vi "TCPReadU8.vi"(8 "error in (no error)":errorcluster, 9 "timeout ms (25000)":i32=25000, 10 "command":string, 11 "connection ID":refnum<k5>) -> (0 "error out":errorcluster, 2 "U8 value":u8, 3 "connection ID out":refnum<k5>)   [LabVIEW 2013]
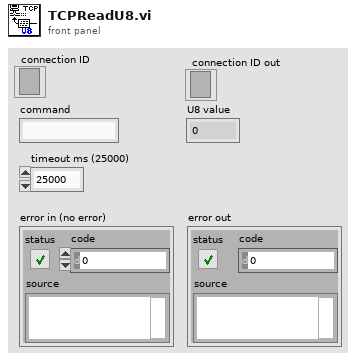
[diagram p1: front panel]
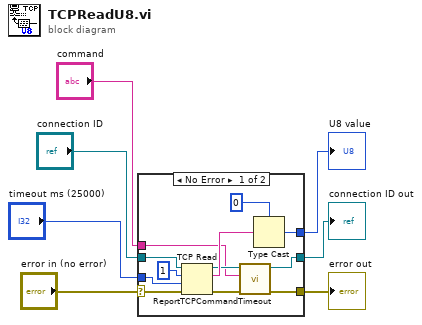
[diagram p0: block diagram]
diagram:
  n1 = case shown="No Error" "error in (no error)" {
    selector: "error in (no error)" -> [w8 w20]
    tunnel: "connection ID" -> [w15 w21]
    tunnel: "command" -> [w14 _]
    tunnel: "timeout ms (25000)" -> [w13 _]
    tunnel: [w12 w20] -> w4
    tunnel: [w11 w21] -> w3
    tunnel: [w10 _] -> w2
    frame No Error {
      n2 = TCP Read(connection ID=w15, bytes to read=1, error in (no error)=w8, 9:w13) -> (connection ID out=w16:refnum<k5>, data out=w19:string, error out=w17:errorcluster)  [unwired: 1 in]
      n3 = call "ReportTCPCommandTimeout.vi"("error in (no error)"=w17, "command"=w14, "connection ID"=w16) -> ("error out"=w12:errorcluster, "connection ID out"=w11:refnum<k5>)  [unwired: 7 in]
      n4 = Type Cast(type=u8 0 ("U8 value"), x=w19) -> (*(type *) &x=w10:u8)
    }
    frame Error {
    }
  }
  "connection ID out" <- w3
  "error out" <- w4
  "U8 value" <- w2
